vi "max value.vi"(7 "unit":string, 8 "error in (no error)":errorcluster, 10 "waveform in":waveform(dbl), 11 "Raw refum":refnum<vi>) -> (0 "error out":errorcluster, 2 "Pmax":string, 3 "引用输出":refnum<vi>)   [LabVIEW 2011]
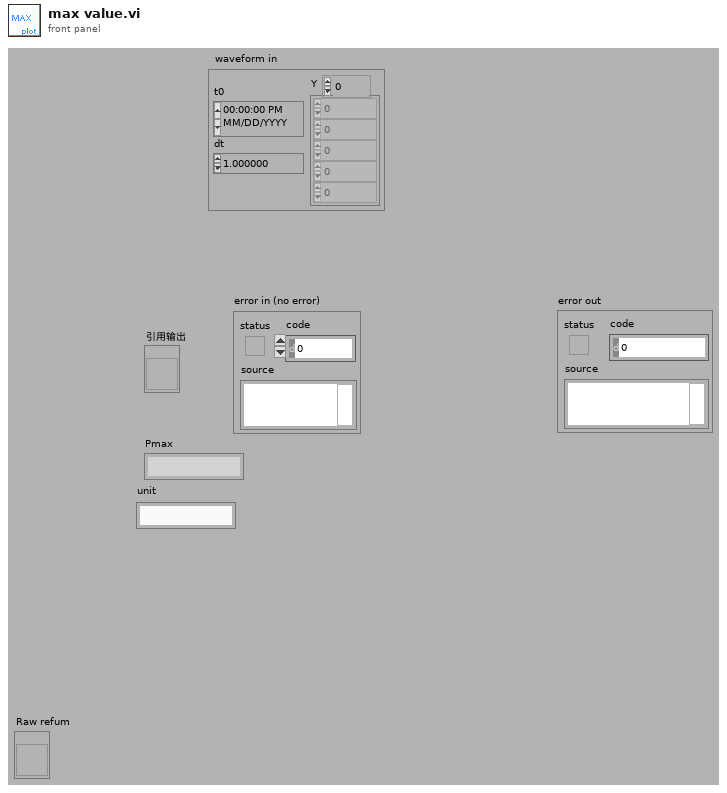
[diagram p1: front panel]
types:
  T1 = enum16{"User-specified Font", "Application Font", "System Font", "Dialog Font"}
  T2 = typedef "LVRectTypeDef.ctl" = cluster{"left":i16, "top":i16, "right":i16, "bottom":i16}
  T3 = typedef "LVPoint32TypeDef.ctl" = cluster{"Horizontal":i32, "Vertical":i32}
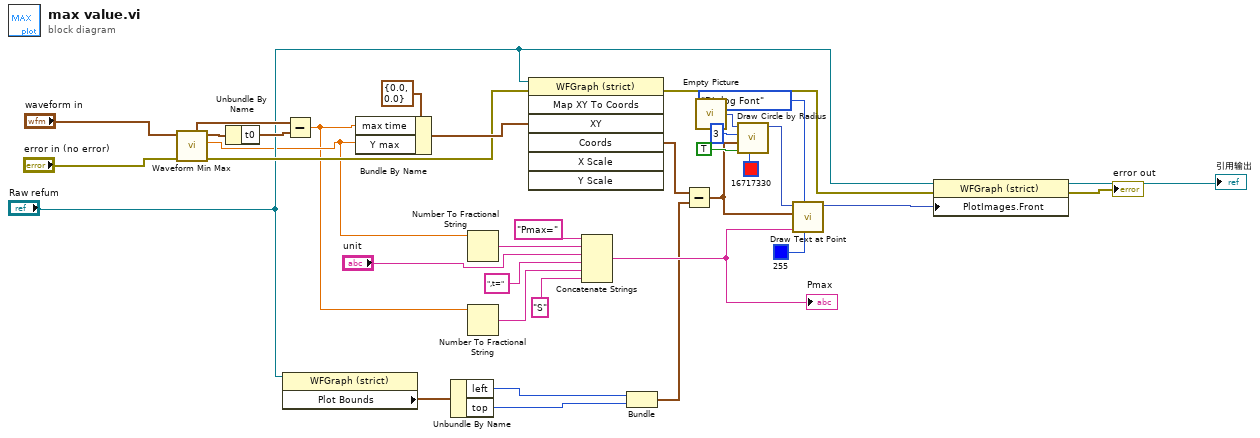
[diagram p0: block diagram]
diagram:
  n1 = call <vilib>:"Waveform Min Max.vi"("error in (no error)"="error in (no error)", "waveform in"="waveform in") -> ("error out"=w8:errorcluster, "Y max"=w2:dbl, "waveform out"=w32:waveform(dbl), "max time"=w34:timestamp)  [unwired: 6 out]
  n2 = Unbundle By Name(w32) -> ("t0"=w33:timestamp)
  n3 = property on="Property Node" class="WFGraph (strict)"(reference="Raw refum") -> ("Plot Bounds"=w14:T2)  [unwired: 1 in, 2 out]
  n4 = Subtract(x=w34, y=w33) -> (x-y=w1:dbl)
  n5 = Bundle By Name(cluster=cluster{"max time":dbl, "Y max":dbl} {"max time"=0.0, "Y max"=0.0}, "max time"=w1, "Y max"=w2) -> (w11:cluster{"max time":dbl, "Y max":dbl})
  n6 = Unbundle By Name(w14) -> ("left"=w15:i16, "top"=w16:i16)
  n7 = Number To Fractional String(number=w2) -> (F-format string=w24:string)  [unwired: 3 out]
  n8 = Number To Fractional String(number=w1) -> (F-format string=w23:string)  [unwired: 3 out]
  n9 = invoke class="WFGraph (strict)" method="Map XY To Coords"(reference="Raw refum", error in=w8, "XY"=w11) -> (error out=w9:errorcluster, "Coords"=w13:T3)  [unwired: 4 in, 5 out]
  n10 = Concatenate Strings("Pmax=", w24, "unit", ",t=" ("string"), w23, "S" ("string")) -> (w21:string)
  "Pmax" <- w21
  n11 = Bundle("left"=w15, "top"=w16) -> (w17:cluster{"left":i16, "top":i16})  [unwired: 1 out]
  n12 = Subtract(x=w13, y=w17) -> (x-y=w12:T3)
  n13 = call "Empty Picture"() -> ("empty picture"=w29:picture)
  n14 = call <vilib>:"Draw Circle by Radius.vi"("color(black)"=u32 16717330, "fill?(F)"=TRUE, "pixel center"=w12, "radius"=i16 3, "picture"=w29) -> ("new picture"=w27:picture)  [unwired: 3 in, 3 out]
  n15 = call <vilib>:"Draw Text at Point.vi"("text color(black)"=u32 255, "desired font(Application)"=T1."Dialog Font", "text"=w21, "origin"=w12, "picture"=w27) -> ("new picture"=w26:picture)  [unwired: 4 in, 2 out]
  n16 = property class="WFGraph (strict)"(reference="Raw refum", error in=w9, "PlotImages.Front"=w26) -> (reference out=→"引用输出":refnum<vi>, error out=→"error out":errorcluster)
